vi "User InterfaceSam.vi"() -> ()   [LabVIEW 2014]
uses:
  controls/Control ConfigurationSam.ctl
  controls/Control StateSam.ctl
  <vilib>/robotics/Controls/Compass Indicator/Compass Indicator.xctl
  controls/UI DataSam.ctl
  globals/UI Network Stream EndpointsSam.vi
panel:
  in  "Run Control 1":bool
  in  "Stop Control 1":bool
  in  "Exit":bool
  out "Current Control Mode":T1
  out "System Status":string
  in  "Settings Tab":T2(tab)
  in  "Compass Control Configuration":T3={"PID Gains"={"proportional gain (Kc)"=1.0, "integral gain (Kc*Ts/Ti)"=0.1, "derivative gain (Kc*Td/Ts)"=0.0}}
  out "Gauge":dbl(knob)=0.028871329670917018 scale=0.0..360.0
  out "Compass Indicator":dbl(xcontrol)
  out "Compass Heading":dbl
  in  "Update Control Configuration 5":bool
  out "Speed Motor 1 Values":cluster{"Double":dbl, "Channel 0 Setpoint":dbl}(graph)
  in  "Motor 1 Setpoint":dbl
  out "Speed Motor 2 Values":cluster{"Double":dbl, "Channel 0 Setpoint":dbl}(graph)
  in  "Motor 2 Setpoint":dbl
  in  "Motor 4 Setpoint":dbl
  out "Speed Motor 4 Values":cluster{i16, "Motor 4 Setpoint":dbl}(graph)
  out "Speed Motor 3 Values":cluster{i16, "Motor 3 Setpoint":dbl}(graph)
  in  "Motor 3 Setpoint":dbl
  in  "Control Configurations 1":T3={"PID Gains"={"proportional gain (Kc)"=2.8, "integral gain (Kc*Ts/Ti)"=1.5, "derivative gain (Kc*Td/Ts)"=0.01}}
  in  "Update Control Configuration 1":bool
  in  "Control Configurations 2":T3={"PID Gains"={"proportional gain (Kc)"=2.8, "integral gain (Kc*Ts/Ti)"=1.5, "derivative gain (Kc*Td/Ts)"=0.01}}
  in  "Update Control Configuration 2":bool
  in  "Control Configurations 3":T3={"PID Gains"={"proportional gain (Kc)"=2.8, "integral gain (Kc*Ts/Ti)"=1.5, "derivative gain (Kc*Td/Ts)"=0.01}}
  in  "Update Control Configuration 3":bool
  in  "Control Configurations 4":T3={"PID Gains"={"proportional gain (Kc)"=2.8, "integral gain (Kc*Ts/Ti)"=1.5, "derivative gain (Kc*Td/Ts)"=0.01}}
  in  "Update Control Configuration 4":bool
  out "Free memory Memory (bytes)":dbl(graph)
  out "CPU Usage (%)":dbl(graph)
  out "Connected?":bool
  in  "Connect to Controller":bool
  in  "Controller Address":string="172.16.0.1"
  # "MyRIO Robot"
  # "Connection Settings"
  # "Degrees"
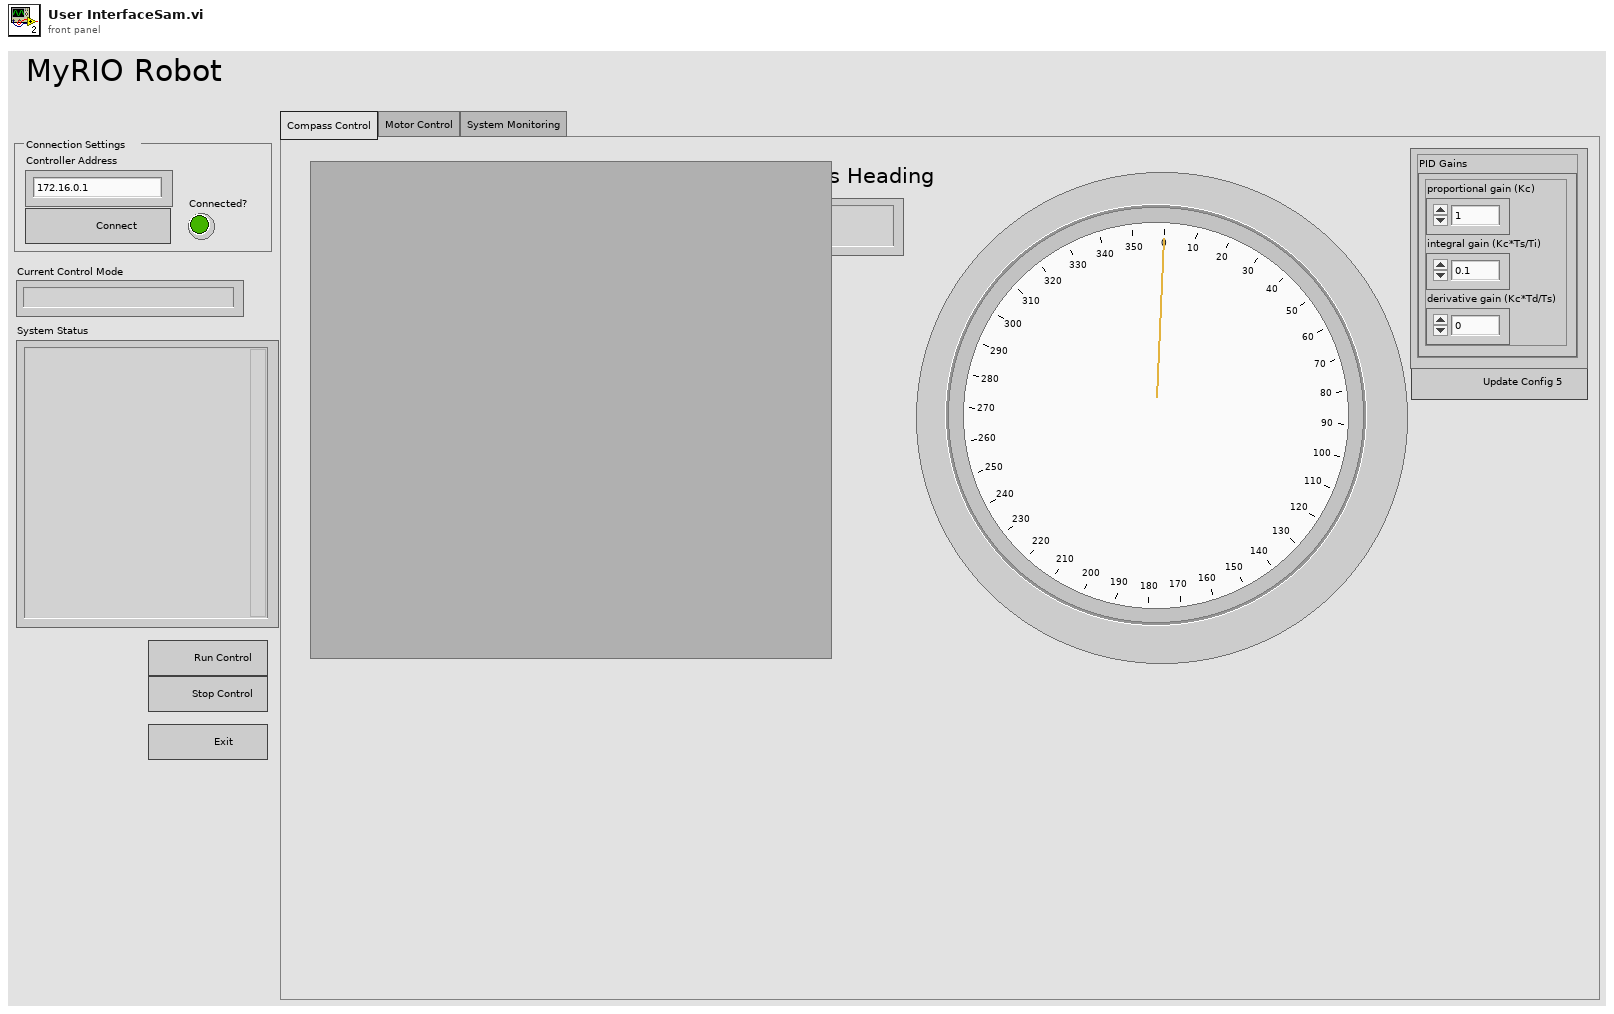
[diagram p1: front panel]
types:
  T1 = typedef "Control StateSam.ctl" = enum16{"", "Control State (PID)", "Safe State"}
  T2 = enum32{"Compass Control", "Motor Control", "System Monitoring"}
  T3 = typedef "Control ConfigurationSam.ctl" = cluster{"PID Gains":cluster{"proportional gain (Kc)":dbl, "integral gain (Kc*Ts/Ti)":dbl, "derivative gain (Kc*Td/Ts)":dbl}}
  T4 = typedef "UI DataSam.ctl" = cluster{"Message":string, "Data":variant}
  T5 = typedef "UI Data.ctl" = cluster{"Message":string, "Data":variant}
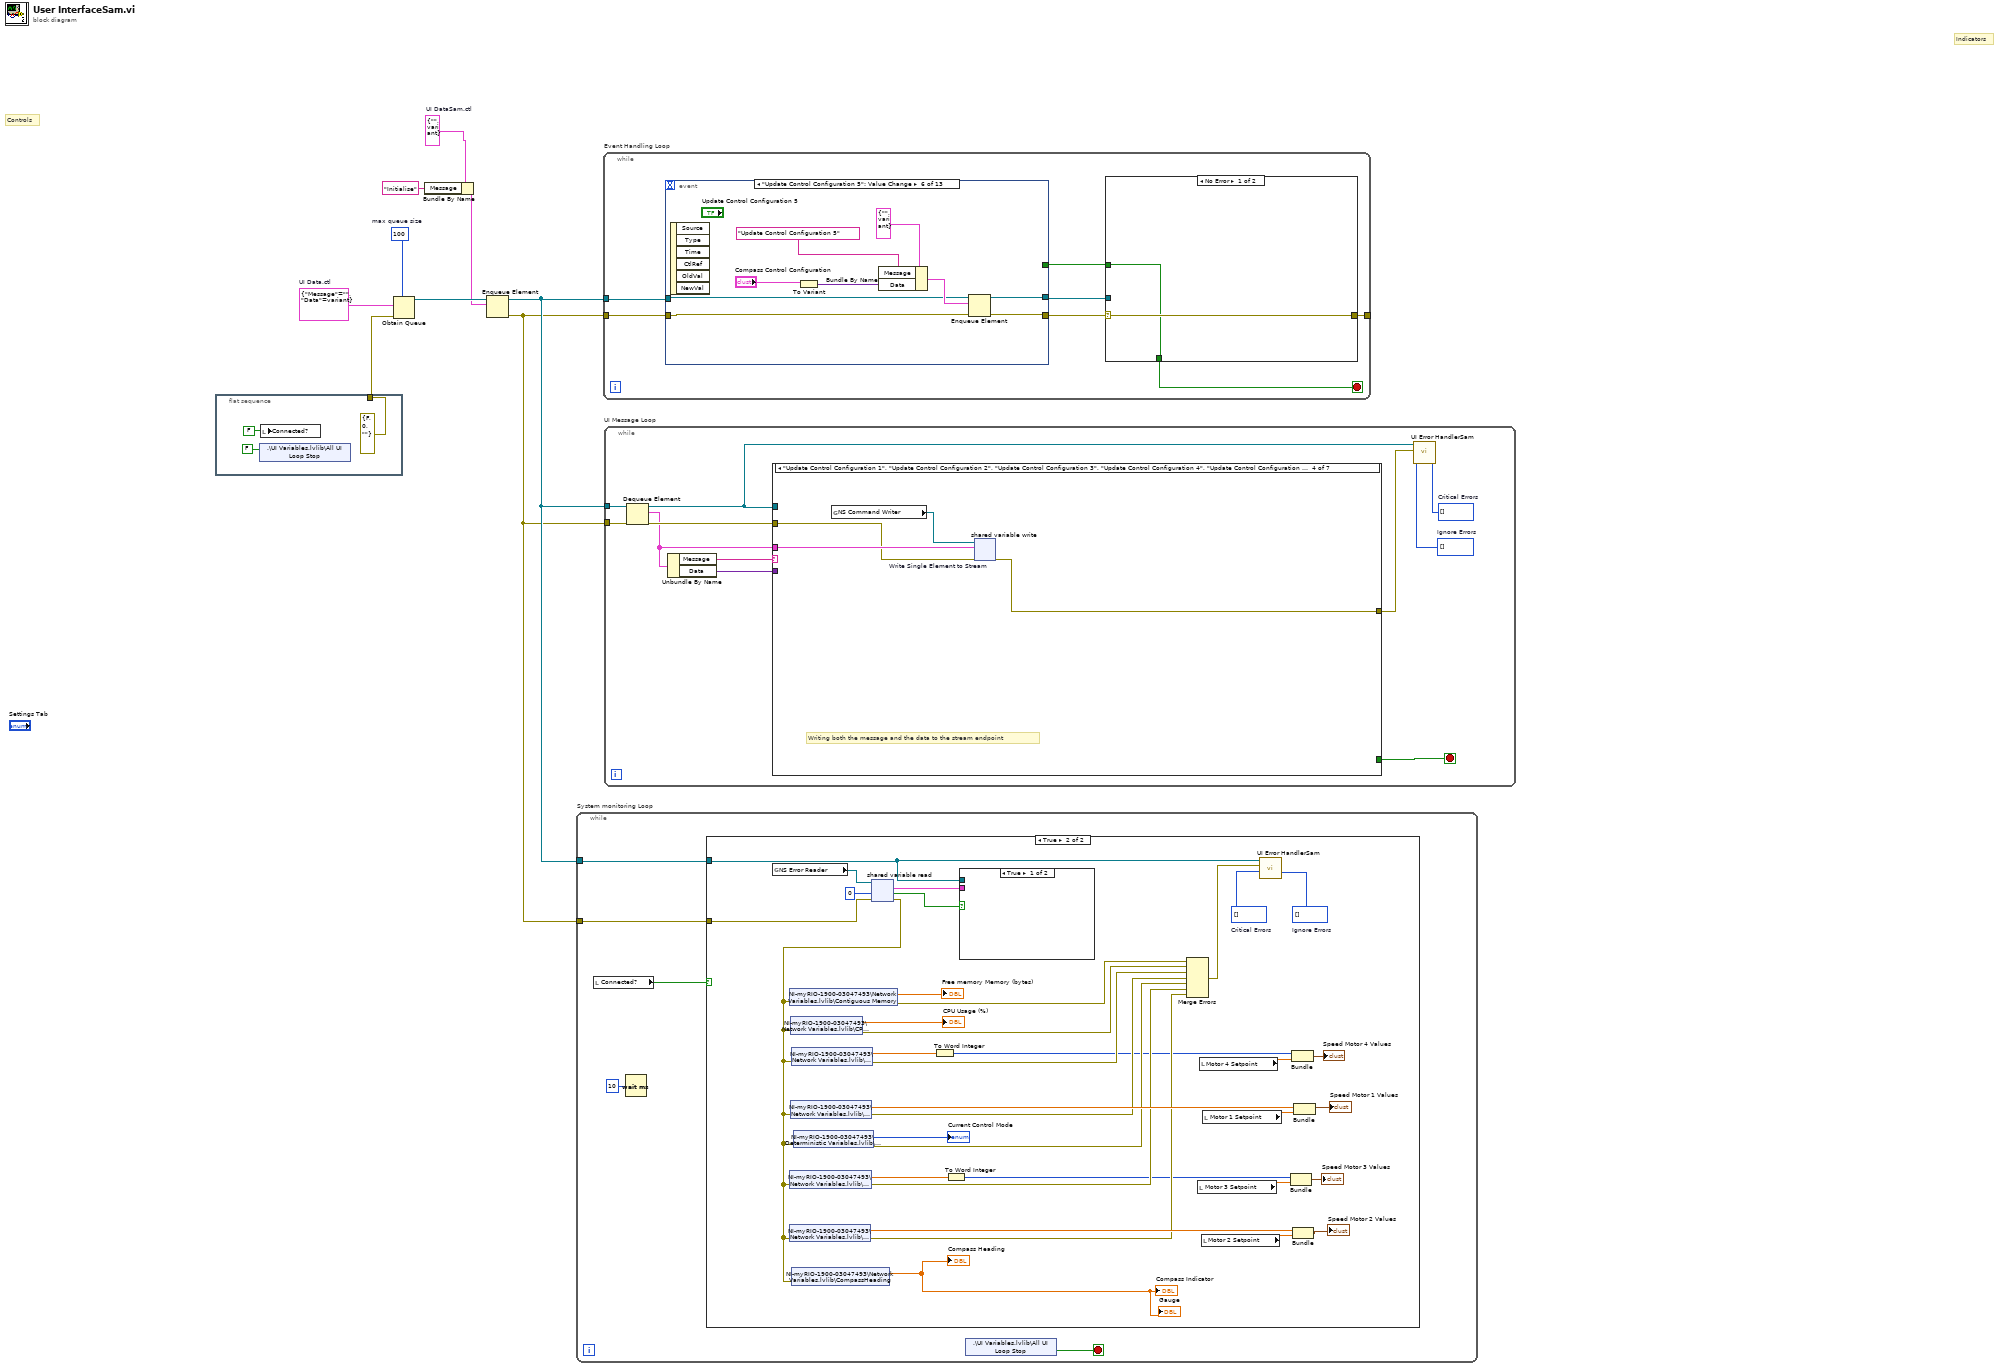
[diagram p0: block diagram]
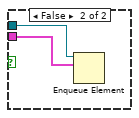
[diagram p3: hidden frame]
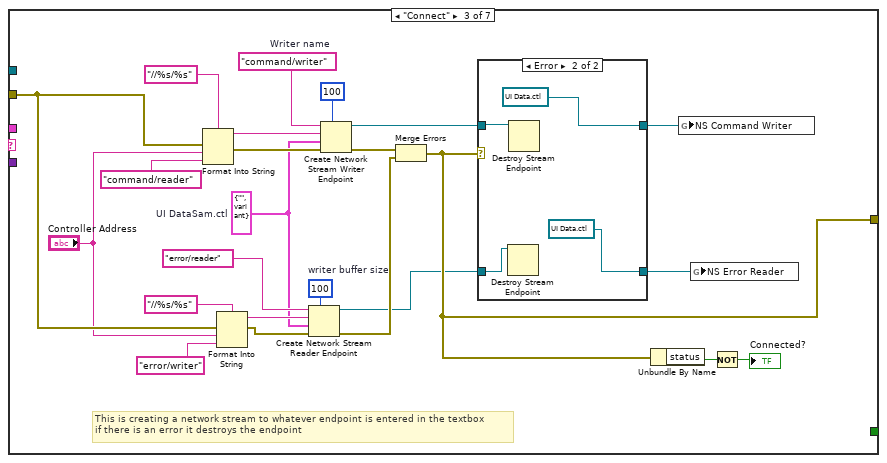
[diagram p6: hidden frame]
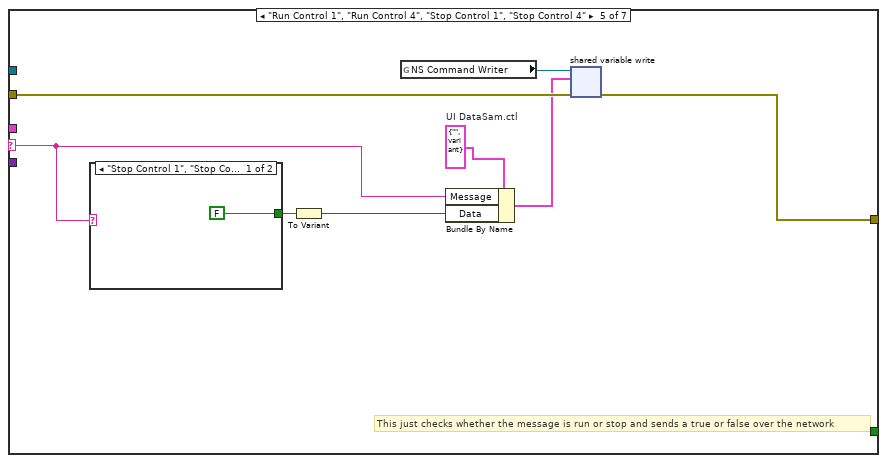
[diagram p8: hidden frame]
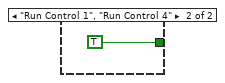
[diagram p9: hidden frame]
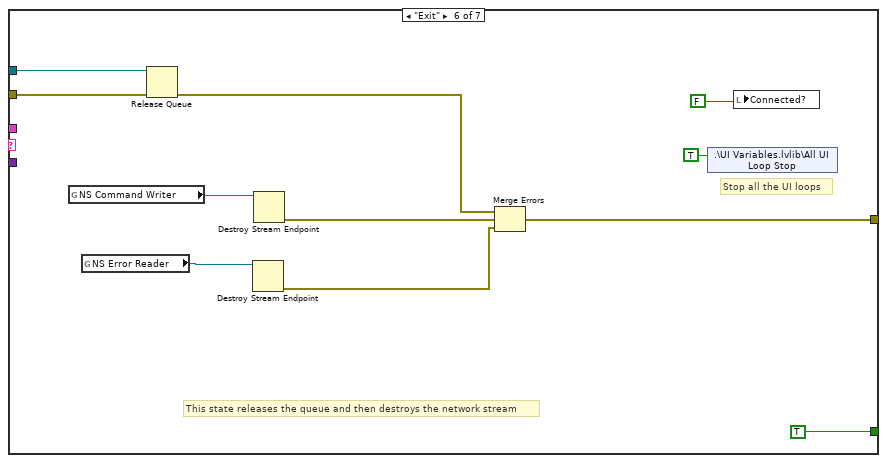
[diagram p10: hidden frame]
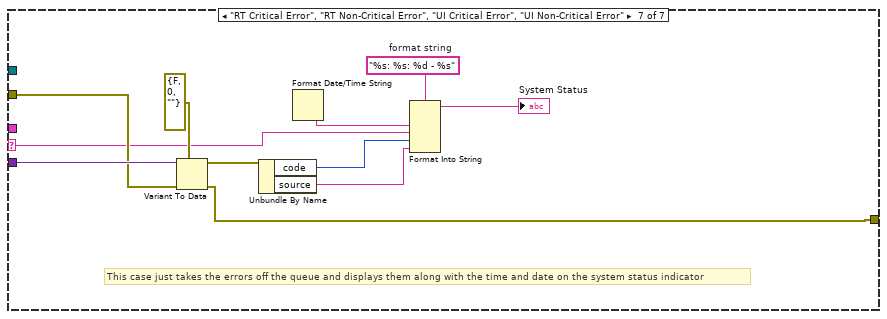
[diagram p11: hidden frame]
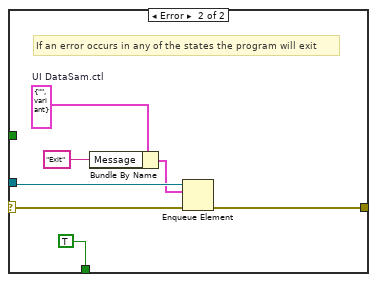
[diagram p12: hidden frame]
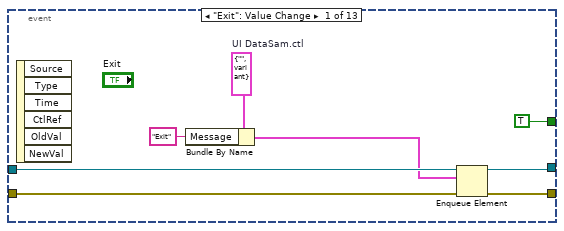
[diagram p13: hidden frame]
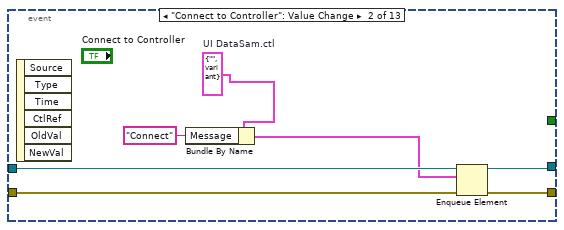
[diagram p14: hidden frame]
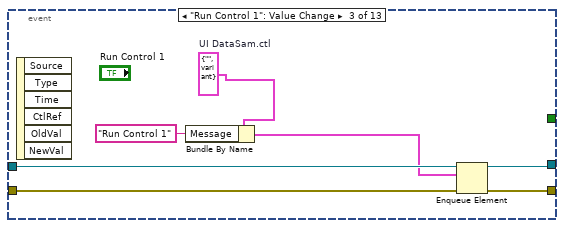
[diagram p15: hidden frame]
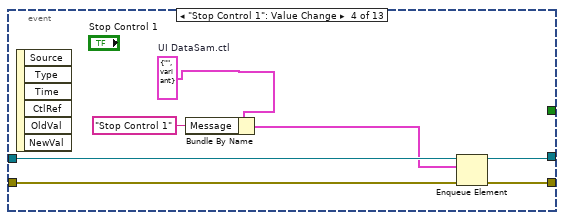
[diagram p16: hidden frame]
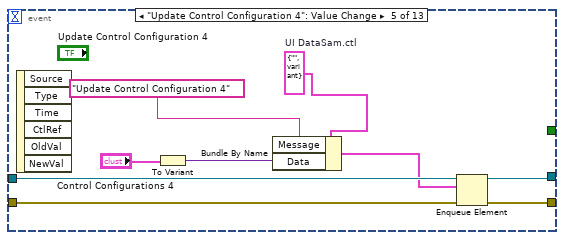
[diagram p17: hidden frame]
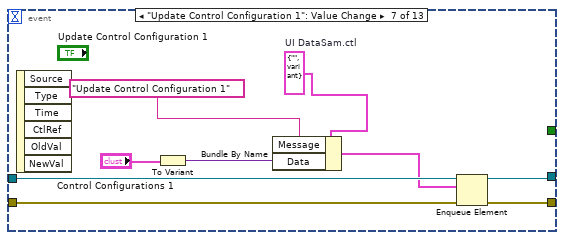
[diagram p18: hidden frame]
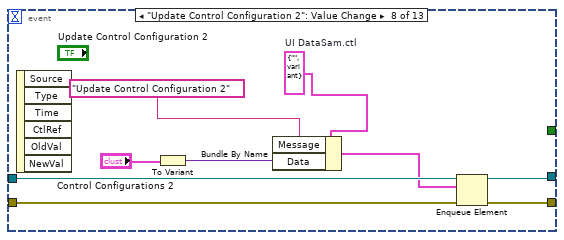
[diagram p19: hidden frame]
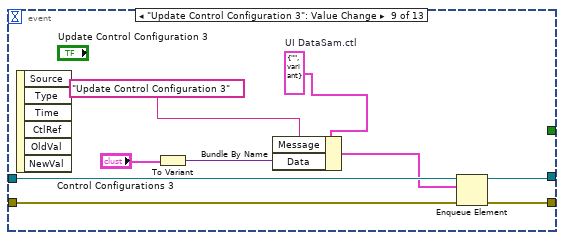
[diagram p20: hidden frame]
diagram:
  w2 = T4 {"Message"="", "Data"=variant}  # UI DataSam.ctl
  w5 = T4 {"Message"="", "Data"=variant}  # UI Data.ctl
  w8 = 100  # max queue size
  # "Indicators"
  # "Controls"
  n1 = flat-sequence {
    tunnel: [w11] -> _
    tunnel: [w11] -> w4
    frame #0 {
      w11 = errorcluster {"status"=FALSE, "code"=0, "source"=""} ("error in (no error)")
      n2 = shared-variable ".\\UI Variables.lvlib\\All UI Loop Stop"(FALSE ("All UI Loop Stop")) -> ()  [unwired: 1 in, 1 out]
      n3 = local write "Connected?"(FALSE ("Connected?")) -> ()
    }
  }
  n4 = Obtain Queue(max queue size (-1, unlimited)=w8, element data type=w5, error in (no error)=w4) -> (queue out=w9:refnum<queue>)  [unwired: 2 in, 2 out]
  n5 = Bundle By Name(cluster=w2, "Message"="Initialise") -> (w6:T4)
  n6 = Enqueue Element(queue=w9, element=w6) -> (queue out=w3:refnum<queue>, error out=w1:errorcluster)  [unwired: 2 in, 1 out]
  n7 = while "System monitoring Loop" {
    tunnel: w3 -> [w14]
    tunnel: w1 -> [w13]
    stop <- w15 stop-if-true
    n8 = local read "Connected?"() -> (w17:bool)
    n9 = Wait (ms)(milliseconds to wait=u32 10) -> ()  [unwired: 1 out]
    n10 = case shown="True" w17 {
      tunnel: w14 -> [_ w42]
      tunnel: w13 -> [_ w39]
      frame False {
      }
      frame True {
        w40 = i32[] []  # Ignore Errors
        w41 = i32[] []  # Critical Errors
        n11 = global read "UI Network Stream EndpointsSam.vi" "NS Error Reader"() -> (w50:refnum<k21>)
        n12 = shared-variable-read(w50, w39, 0 ("timeout ms (-1)")) -> (w19:errorcluster, w47:bool, w48:T5)  [unwired: 1 out]
        n13 = shared-variable "NI-myRIO-1900-03047493\\Network Variables.lvlib\\Contiguous Memory"(error in=w19) -> (→"Free memory Memory (bytes)":dbl, error out=w44:errorcluster)
        n14 = shared-variable "NI-myRIO-1900-03047493\\Network Variables.lvlib\\SpeedMotor2"(error in=w19) -> (w31:dbl, error out=w24:errorcluster)
        n15 = shared-variable "NI-myRIO-1900-03047493\\Network Variables.lvlib\\SpeedMotor3"(error in=w19) -> (w21:dbl, error out=w25:errorcluster)
        n16 = shared-variable "NI-myRIO-1900-03047493\\Network Variables.lvlib\\CPU Usage"(error in=w19) -> (→"CPU Usage (%)":dbl, error out=w45:errorcluster)
        n17 = shared-variable "NI-myRIO-1900-03047493\\Network Variables.lvlib\\SpeedMotor1"(error in=w19) -> (w35:dbl, error out=w27:errorcluster)
        n18 = shared-variable "NI-myRIO-1900-03047493\\Network Variables.lvlib\\SpeedMotor4"(error in=w19) -> (w23:dbl, error out=w46:errorcluster)
        n19 = shared-variable "NI-myRIO-1900-03047493\\Network Variables.lvlib\\CompassHeading"(error in=w19) -> (→"Compass Heading" →"Compass Indicator" →"Gauge":dbl)  [unwired: 1 out]
        n20 = shared-variable "NI-myRIO-1900-03047493\\Deterministic Variables.lvlib\\Control State"(error in=w19) -> (→"Current Control Mode":T1, error out=w26:errorcluster)
        n21 = To Word Integer(number=w23) -> (16bit integer=w22:i16)
        n22 = To Word Integer(number=w21) -> (16bit integer=w20:i16)
        n23 = case shown="True" w47 {
          tunnel: w48 -> [_ w53]
          tunnel: w42 -> [_ w54]
          frame True {
          }
          frame False {
            n24 = Enqueue Element(queue=w54, element=w53) -> ()  [unwired: 2 in, 3 out]
          }
        }
        n25 = Merge Errors(w44, w45, w46, w27, w26, w25, w24) -> (w43:errorcluster)
        n26 = local read "Motor 3 Setpoint"() -> (w28:dbl)
        n27 = local read "Motor 4 Setpoint"() -> (w38:dbl)
        n28 = local read "Motor 2 Setpoint"() -> (w30:dbl)
        n29 = local read "Motor 1 Setpoint"() -> (w36:dbl)
        n30 = call "UI Error HandlerSam.vi"("Ignore Errors"=w40, "Critical Errors"=w41, "error to process"=w43, "queue in"=w42) -> ()  [unwired: 7 in, 1 out]
        n31 = Bundle(w20, "Motor 3 Setpoint"=w28) -> (→"Speed Motor 3 Values":cluster{i16, "Motor 3 Setpoint":dbl})  [unwired: 1 in]
        n32 = Bundle(w22, "Motor 4 Setpoint"=w38) -> (→"Speed Motor 4 Values":cluster{i16, "Motor 4 Setpoint":dbl})  [unwired: 1 in]
        n33 = Bundle("Double"=w31, "Motor 2 Setpoint"=w30) -> (→"Speed Motor 2 Values":cluster{"Double":dbl, "Motor 2 Setpoint":dbl})  [unwired: 1 in]
        n34 = Bundle("Double"=w35, "Motor 1 Setpoint"=w36) -> (→"Speed Motor 1 Values":cluster{"Double":dbl, "Motor 1 Setpoint":dbl})  [unwired: 1 in]
      }
    }
    n35 = shared-variable ".\\UI Variables.lvlib\\All UI Loop Stop"() -> (w15:bool)  [unwired: 1 in, 1 out]
  }
  n36 = while "Event Handling Loop" {
    tunnel: w3 -> [w61]
    tunnel: w1 -> [w60]
    tunnel: [w56] -> _
    stop <- w55 stop-if-true
    n37 = event shown="[5] \"Update Control Configuration 5\": Value Change" {
      selector: _ -> [_ _ _ _ _ _ _ _ _ _ _ _ _]
      dyn-events: _ -> [_ _ _ _ _ _ _ _ _ _ _ _ _]
      timeout: _ -> [_ _ _ _ _ _ _ _ _ _ _ _ _]
      tunnel: w61 -> [w77 w84 w91 w98 w107 w110 w125 w134 w143 w152 w161 w170 w179]
      tunnel: w60 -> [w76 w83 w90 w97 w106 w109 w124 w133 w142 w151 w160 w169 w178]
      tunnel: [w74 w81 w88 w95 w104 w113 w122 w131 w140 w149 w158 w167 w176] -> w58
      tunnel: [w73 w80 w87 w94 w103 w112 w121 w130 w139 w148 w157 w166 w175] -> w59
      tunnel: [TRUE _ _ _ _ _ _ _ _ _ _ _ _] -> w57
      event "Exit": Value Change {
        w71 = T4 {"Message"="", "Data"=variant}  # UI DataSam.ctl
        n38 = event-data() -> ()  [unwired: 1 in, 6 out]
        n39 = Bundle By Name(cluster=w71, "Message"="Exit") -> (w75:T4)
        n40 = Enqueue Element(queue=w77, element=w75, error in (no error)=w76) -> (queue out=w74:refnum<queue>, error out=w73:errorcluster)  [unwired: 1 in, 1 out]
      }
      event "Connect to Controller": Value Change {
        w79 = T4 {"Message"="", "Data"=variant}  # UI DataSam.ctl
        n41 = event-data() -> ()  [unwired: 1 in, 6 out]
        n42 = Bundle By Name(cluster=w79, "Message"="Connect") -> (w82:T4)
        n43 = Enqueue Element(queue=w84, element=w82, error in (no error)=w83) -> (queue out=w81:refnum<queue>, error out=w80:errorcluster)  [unwired: 1 in, 1 out]
      }
      event "Run Control 1": Value Change {
        w86 = T4 {"Message"="", "Data"=variant}  # UI DataSam.ctl
        n44 = event-data() -> ()  [unwired: 1 in, 6 out]
        n45 = Bundle By Name(cluster=w86, "Message"="Run Control 1") -> (w89:T4)
        n46 = Enqueue Element(queue=w91, element=w89, error in (no error)=w90) -> (queue out=w88:refnum<queue>, error out=w87:errorcluster)  [unwired: 1 in, 1 out]
      }
      event "Stop Control 1": Value Change {
        w93 = T4 {"Message"="", "Data"=variant}  # UI DataSam.ctl
        n47 = event-data() -> ()  [unwired: 1 in, 6 out]
        n48 = Bundle By Name(cluster=w93, "Message"="Stop Control 1") -> (w96:T4)
        n49 = Enqueue Element(queue=w98, element=w96, error in (no error)=w97) -> (queue out=w95:refnum<queue>, error out=w94:errorcluster)  [unwired: 1 in, 1 out]
      }
      event "Update Control Configuration 4": Value Change {
        w100 = T4 {"Message"="", "Data"=variant}  # UI DataSam.ctl
        n50 = event-data() -> ()  [unwired: 1 in, 6 out]
        n51 = To Variant(anything="Control Configurations 4") -> (Variant=w101:variant)
        n52 = Bundle By Name(cluster=w100, "Message"="Update Control Configuration 4", "Data"=w101) -> (w105:T4)
        n53 = Enqueue Element(queue=w107, element=w105, error in (no error)=w106) -> (queue out=w104:refnum<queue>, error out=w103:errorcluster)  [unwired: 1 in, 1 out]
      }
      event "Update Control Configuration 5": Value Change {
        n54 = event-data() -> ()  [unwired: 1 in, 6 out]
        n55 = To Variant(anything="Compass Control Configuration") -> (Variant=w116:variant)
        n56 = Bundle By Name(cluster=T4 {"Message"="", "Data"=variant} ("Cluster"), "Message"="Update Control Configuration 5", "Data"=w116) -> (w111:T4)
        n57 = Enqueue Element(queue=w110, element=w111, error in (no error)=w109) -> (queue out=w113:refnum<queue>, error out=w112:errorcluster)  [unwired: 1 in, 1 out]
      }
      event "Update Control Configuration 1": Value Change {
        w118 = T4 {"Message"="", "Data"=variant}  # UI DataSam.ctl
        n58 = event-data() -> ()  [unwired: 1 in, 6 out]
        n59 = To Variant(anything="Control Configurations 1") -> (Variant=w119:variant)
        n60 = Bundle By Name(cluster=w118, "Message"="Update Control Configuration 1", "Data"=w119) -> (w123:T4)
        n61 = Enqueue Element(queue=w125, element=w123, error in (no error)=w124) -> (queue out=w122:refnum<queue>, error out=w121:errorcluster)  [unwired: 1 in, 1 out]
      }
      event "Update Control Configuration 2": Value Change {
        w127 = T4 {"Message"="", "Data"=variant}  # UI DataSam.ctl
        n62 = event-data() -> ()  [unwired: 1 in, 6 out]
        n63 = To Variant(anything="Control Configurations 2") -> (Variant=w128:variant)
        n64 = Bundle By Name(cluster=w127, "Message"="Update Control Configuration 2", "Data"=w128) -> (w132:T4)
        n65 = Enqueue Element(queue=w134, element=w132, error in (no error)=w133) -> (queue out=w131:refnum<queue>, error out=w130:errorcluster)  [unwired: 1 in, 1 out]
      }
      event "Update Control Configuration 3": Value Change {
        w136 = T4 {"Message"="", "Data"=variant}  # UI DataSam.ctl
        n66 = event-data() -> ()  [unwired: 1 in, 6 out]
        n67 = To Variant(anything="Control Configurations 3") -> (Variant=w137:variant)
        n68 = Bundle By Name(cluster=w136, "Message"="Update Control Configuration 3", "Data"=w137) -> (w141:T4)
        n69 = Enqueue Element(queue=w143, element=w141, error in (no error)=w142) -> (queue out=w140:refnum<queue>, error out=w139:errorcluster)  [unwired: 1 in, 1 out]
      }
      event "Motor 4 Setpoint": Value Change {
        w145 = T4 {"Message"="", "Data"=variant}  # UI DataSam.ctl
        n70 = event-data() -> ()  [unwired: 1 in, 6 out]
        n71 = To Variant(anything="Motor 4 Setpoint") -> (Variant=w147:variant)
        n72 = Bundle By Name(cluster=w145, "Message"="Update Motor 4 Setpoint", "Data"=w147) -> (w150:T4)
        n73 = Enqueue Element(queue=w152, element=w150, error in (no error)=w151) -> (queue out=w149:refnum<queue>, error out=w148:errorcluster)  [unwired: 1 in, 1 out]
      }
      event "Motor 2 Setpoint": Value Change {
        w154 = T4 {"Message"="", "Data"=variant}  # UI DataSam.ctl
        n74 = event-data() -> ()  [unwired: 1 in, 6 out]
        n75 = To Variant(anything="Motor 2 Setpoint") -> (Variant=w156:variant)
        n76 = Bundle By Name(cluster=w154, "Message"="Update Motor 2 Setpoint", "Data"=w156) -> (w159:T4)
        n77 = Enqueue Element(queue=w161, element=w159, error in (no error)=w160) -> (queue out=w158:refnum<queue>, error out=w157:errorcluster)  [unwired: 1 in, 1 out]
      }
      event "Motor 3 Setpoint": Value Change {
        w163 = T4 {"Message"="", "Data"=variant}  # UI DataSam.ctl
        n78 = event-data() -> ()  [unwired: 1 in, 6 out]
        n79 = To Variant(anything="Motor 3 Setpoint") -> (Variant=w165:variant)
        n80 = Bundle By Name(cluster=w163, "Message"="Update Motor 3 Setpoint", "Data"=w165) -> (w168:T4)
        n81 = Enqueue Element(queue=w170, element=w168, error in (no error)=w169) -> (queue out=w167:refnum<queue>, error out=w166:errorcluster)  [unwired: 1 in, 1 out]
      }
      event "Motor 1 Setpoint": Value Change {
        w173 = T4 {"Message"="", "Data"=variant}  # UI DataSam.ctl
        n82 = event-data() -> ()  [unwired: 1 in, 6 out]
        n83 = To Variant(anything="Motor 1 Setpoint") -> (Variant=w174:variant)
        n84 = Bundle By Name(cluster=w173, "Message"="Update Motor 1 Setpoint", "Data"=w174) -> (w177:T4)
        n85 = Enqueue Element(queue=w179, element=w177, error in (no error)=w178) -> (queue out=w176:refnum<queue>, error out=w175:errorcluster)  [unwired: 1 in, 1 out]
      }
    }
    n86 = case shown="No Error" w59 {
      selector: w59 -> [w63 w68]
      tunnel: w58 -> [_ w69]
      tunnel: w57 -> [w62 _]
      tunnel: [w63 w66] -> w56
      tunnel: [w62 TRUE] -> w55
      frame No Error {
      }
      frame Error {
        w64 = T4 {"Message"="", "Data"=variant}  # UI DataSam.ctl
        # "If an error occurs in any of the states the program will exit"
        n87 = Bundle By Name(cluster=w64, "Message"="Exit") -> (w67:T4)
        n88 = Enqueue Element(queue=w69, element=w67, error in (no error)=w68) -> (error out=w66:errorcluster)  [unwired: 1 in, 2 out]
      }
    }
  }
  n89 = while "UI Message Loop" {
    tunnel: w3 -> [w191]
    tunnel: w1 -> [w190]
    stop <- w187 stop-if-true
    w182 = i32[] []  # Ignore Errors
    w183 = i32[] []  # Critical Errors
    n90 = Dequeue Element(queue=w191, error in (no error)=w190) -> (queue out=w185:refnum<queue>, element=w186:T4, error out=w188:errorcluster)  [unwired: 1 in, 1 out]
    n91 = Unbundle By Name(w186) -> ("Message"=w189:string, "Data"=w181:variant)
    n92 = case shown="\"Update Control Configuration 1\", \"Update Control Configuration 2\", \"Update Control Configuration 3\", \"Update Control Configuration 4\", \"Update Control Configuration 5\", \"Update Motor 1 Setpoint\", \"Update Motor 2 Setpoint\", \"Update Motor 3 Setpoint\", \"Update Motor 4 Setpoint\"" w189 {
      selector: w189 -> [_ _ _ _ w233 _ w253]
      tunnel: w185 -> [_ _ _ _ _ w247 _]
      tunnel: w188 -> [w192 w193 w201 w224 w232 w246 w258]
      tunnel: [w192 w193 w207 w227 w229 w243 w249] -> w184
      tunnel: [_ _ _ _ _ TRUE _] -> w187
      tunnel: w186 -> [_ _ _ w225 _ _ _]
      tunnel: w181 -> [_ _ _ _ _ _ w259]
      frame "Default", Default {
      }
      frame "Initialise" {
      }
      frame "Connect" {
        w194 = T4 {"Message"="", "Data"=variant}  # UI DataSam.ctl
        w204 = 100  # writer buffer size
        w212 = "command/writer"  # Writer name
        # "This is creating a network stream to whatever endpoint is entered in the textbox\nif there is an error it destroys the endpoint"
        n93 = Format Into String(format string="//%s/%s", error in=w201, "Controller Address", "command/reader" ("input 2")) -> (resulting string=w214:string, error out=w215:errorcluster)  [unwired: 1 in]
        n94 = Format Into String "Format Into String"(format string="//%s/%s", error in=w201, "Controller Address", "error/writer" ("input 2")) -> (resulting string=w203:string, error out=w202:errorcluster)  [unwired: 1 in]
        n95 = Create Network Stream Reader Endpoint(7:w204, 8:w202, 9:w194, 10:w203, 11:"error/reader" ("writer name")) -> (0:w198:errorcluster, 3:w197:refnum<k21>)  [unwired: 2 in]
        n96 = Create Network Stream Writer Endpoint(7:100 ("writer buffer size"), 8:w215, 9:w194, 10:w214, 11:w212) -> (0:w208:errorcluster, 3:w211:refnum<k21>)  [unwired: 2 in]
        n97 = Merge Errors(w208, w198) -> (w207:errorcluster)
        n98 = case shown="Error" w207 {
          tunnel: w211 -> [w219 w223]
          tunnel: [w219 refnum<k21> refnum ("Writer name")] -> w195
          tunnel: [w218 refnum<k21> refnum ("Writer name")] -> w196
          tunnel: w197 -> [w218 w220]
          frame No Error {
          }
          frame Error {
            n99 = Destroy Stream Endpoint(11:w220) -> ()  [unwired: 1 in, 1 out]
            n100 = Destroy Stream Endpoint(11:w223) -> ()  [unwired: 1 in, 1 out]
          }
        }
        n101 = Unbundle By Name(w207) -> ("status"=w210:bool)
        n102 = global write "UI Network Stream EndpointsSam.vi" "NS Command Writer"(w195) -> ()
        n103 = global write "UI Network Stream EndpointsSam.vi" "NS Error Reader"(w196) -> ()
        n104 = Not(x=w210) -> (.not. x?=→"Connected?":bool)
      }
      frame "Update Control Configuration 1", "Update Control Configuration 2", "Update Control Configuration 3", "Update Control Configuration 4", "Update Control Configuration 5", "Update Motor 1 Setpoint", "Update Motor 2 Setpoint", "Update Motor 3 Setpoint", "Update Motor 4 Setpoint" {
        # "Writing both the message and the data to the stream endpoint"
        n105 = global read "UI Network Stream EndpointsSam.vi" "NS Command Writer"() -> (w226:refnum<k21>)
        n106 = shared-variable-write "Write Single Element to Stream"(w226, w224, w225) -> (w227:errorcluster)  [unwired: 1 in, 2 out]
      }
      frame "Run Control 1", "Run Control 4", "Stop Control 1", "Stop Control 4" {
        w228 = T4 {"Message"="", "Data"=variant}  # UI DataSam.ctl
        # "This just checks whether the message is run or stop and sends a true or false over the network"
        n107 = case shown="\"Stop Control 1\", \"Stop Control 4\", Default" w233 {
          tunnel: [FALSE TRUE] -> w235
          frame "Stop Control 1", "Stop Control 4", Default {
          }
          frame "Run Control 1", "Run Control 4" {
          }
        }
        n108 = To Variant(anything=w235) -> (Variant=w234:variant)
        n109 = global read "UI Network Stream EndpointsSam.vi" "NS Command Writer"() -> (w231:refnum<k21>)
        n110 = Bundle By Name(cluster=w228, "Message"=w233, "Data"=w234) -> (w230:T4)
        n111 = shared-variable-write(w231, w232, w230) -> (w229:errorcluster)  [unwired: 1 in, 2 out]
      }
      frame "Exit" {
        # "Stop all the UI loops"
        # "This state releases the queue and then destroys the network stream"
        n112 = global read "UI Network Stream EndpointsSam.vi" "NS Command Writer"() -> (w245:refnum<k21>)
        n113 = global read "UI Network Stream EndpointsSam.vi" "NS Error Reader"() -> (w239:refnum<k21>)
        n114 = Release Queue(queue=w247, error in (no error)=w246) -> (error out=w244:errorcluster)  [unwired: 1 in, 2 out]
        n115 = Destroy Stream Endpoint(11:w239) -> (0:w238:errorcluster)  [unwired: 1 in]
        n116 = Destroy Stream Endpoint(11:w245) -> (0:w242:errorcluster)  [unwired: 1 in]
        n117 = Merge Errors(w244, w242, w238) -> (w243:errorcluster)
        n118 = shared-variable ".\\UI Variables.lvlib\\All UI Loop Stop"(TRUE ("All UI Loop Stop")) -> ()  [unwired: 1 in, 1 out]
        n119 = local write "Connected?"(FALSE) -> ()
      }
      frame "RT Critical Error", "RT Non-Critical Error", "UI Critical Error", "UI Non-Critical Error" {
        w251 = "%s: %s: %d - %s"  # format string
        # "This case just takes the errors off the queue and displays them along with the time and date on the system status indicator"
        n120 = Variant To Data(error in=w258, type=errorcluster {"status"=FALSE, "code"=0, "source"=""} ("error out"), Variant=w259) -> (data=w256:errorcluster, error out=w249:errorcluster)
        n121 = Unbundle By Name(w256) -> ("code"=w254:i32, "source"=w252:string)
        n122 = Format Date/Time String() -> (date/time string=w255:string)  [unwired: 3 in]
        n123 = Format Into String(format string=w251, w255, w253, w254, w252) -> (resulting string=→"System Status":string)  [unwired: 2 in, 1 out]
      }
    }
    n124 = call "UI Error HandlerSam.vi"("Ignore Errors"=w182, "Critical Errors"=w183, "error to process"=w184, "queue in"=w185) -> ()  [unwired: 7 in, 1 out]
  }
